vi "Remove Step.vi"(11 "Settings UI in":refnum<class "Settings UI.lvclass">) -> (3 "Settings UI out":refnum<class "Settings UI.lvclass">)   [LabVIEW 2020, in "Output Sequencer.lvlib" / "Settings UI.lvclass"]
uses:
  Settings UI.lvclass
  Settings UI.lvclass/Settings UI.ctl
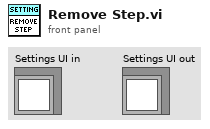
[diagram p1: front panel]
types:
  T1 = map{i32, cluster{"Step Number":i32, "Description":string}}
  T2 = typedef "Output Sequencer.lvlib/Settings UI.lvclass/Step Settings.ctl" = cluster{"Description":string, "Precondition":string, "Duration":dbl, "Mode":string, "Delay Between Values":dbl, "Analog Values":string[], "Digital Values":string[], "Postcondition":string, "On True":string, "On False":string}
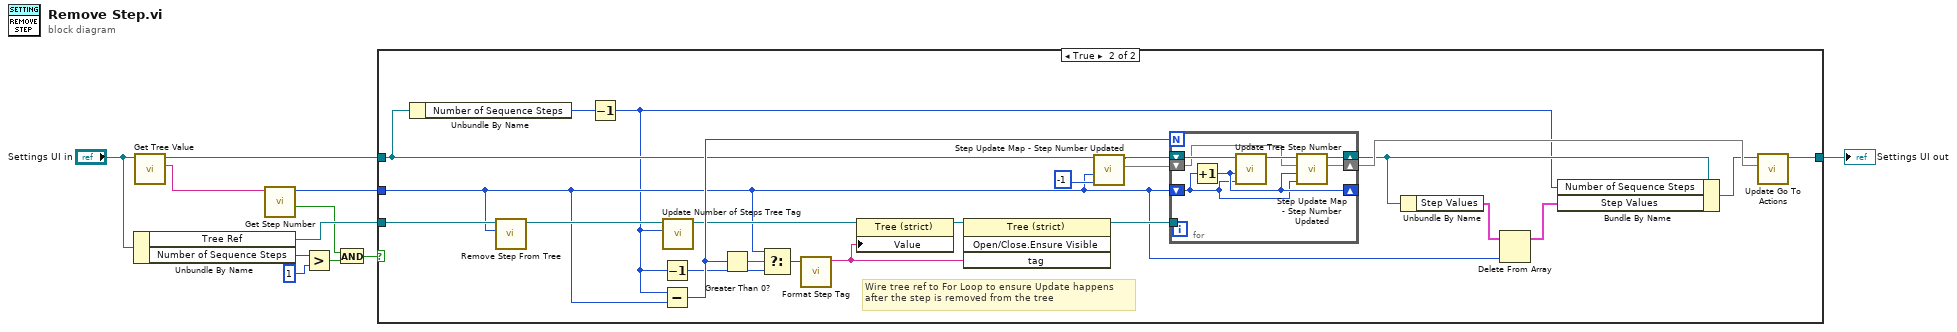
[diagram p0: block diagram]
diagram:
  n1 = Unbundle By Name("Settings UI in") -> ("Tree Ref"=w9:refnum<vi>, "Number of Sequence Steps"=w4:i32)
  n2 = call "Get Tree Value.vi"("UI Data in"="Settings UI in") -> ("Value"=w2:string, "UI Data out"=w10:refnum<class "Settings UI.lvclass">)  [unwired: 9 in]
  n3 = call "Get Step Number.vi"("Tree Tag"=w2) -> ("Is Step tag?"=w7:bool, "Step Number"=w3:i32)  [unwired: 8 in, 1 out]
  n4 = Greater?(x=w4, y=1) -> (0:w6:bool)
  n5 = And(x=w7, y=w6) -> (x .and. y?=w8:bool)
  n6 = case shown="True" w8 {
    tunnel: w3 -> [_ w15]
    tunnel: w10 -> [w12 w14]
    tunnel: [w12 w24] -> w11
    tunnel: w9 -> [_ w27]
    frame False {
    }
    frame True {
      # "Wire tree ref to For Loop to ensure Update happens\nafter the step is removed from the tree"
      n7 = Unbundle By Name(w14) -> ("Number of Sequence Steps"=w35:i32)
      n8 = call "Remove Step From Tree.vi"("Step Index"=w15, "TreeControl in"=w27) -> ("TreeControl out"=w34:refnum<vi>)  [unwired: 9 in]
      n9 = Decrement(x=w35) -> (x-1=w13:i32)
      n10 = Decrement(x=w13) -> (x-1=w31:i32)
      n11 = Subtract(x=w13, y=w15) -> (x-y=w33:i32)
      n12 = call "Update Number of Steps Tree Tag.vi"("New Number of Steps"=w13, "TreeControl in"=w34) -> ("TreeControl out"=w26:refnum<vi>)  [unwired: 9 in]
      n13 = Greater Than 0?(x=w33) -> (x > 0?=w32:bool)
      n14 = Select(t=w15, s=w32, f=w31) -> (s? t:f=w28:i32)
      n15 = call "Format Step Tag.vi"("Step Number"=w28) -> ("Tag"=w29:string)  [unwired: 10 in]
      n16 = property class="Tree (strict)"(reference=w26, "Value"=w29) -> (reference out=w30:refnum<vi>)  [unwired: 1 in, 1 out]
      n17 = invoke class="Tree (strict)" method="Open/Close.Ensure Visible"(reference=w30, "tag"=w29) -> (reference out=w25:refnum<vi>)  [unwired: 2 in, 3 out]
      n18 = call "Step Update Map - Step Number Updated.vi"("New Step Number"=-1, "Previous Step Number"=w15, "Settings UI in"=w14) -> ("Step Update Map out"=w20:T1, "Settings UI out"=w22:refnum<class "Settings UI.lvclass">)  [unwired: 7 in]
      n19 = for {
        N: w33 -> [_]
        shift-right: [w40] -> _
        shift-left: w15 -> [w38]
        shift-right: [w39] -> w19
        shift-left: w22 -> [w42]
        tunnel: w25 -> [_]
        shift-right: [w37] -> w23
        shift-left: w20 -> [w36]
        n20 = Increment(x=w38) -> (x+1=w40:i32)
        n21 = call "Update Tree Step Number.vi"("New Step Number"=w38, "Old Step Number"=w40, "UI Data In"=w42) -> ("UI Data Out"=w41:refnum<class "Settings UI.lvclass">)  [unwired: 6 in, 2 out]
        n22 = call "Step Update Map - Step Number Updated.vi"("New Step Number"=w38, "Previous Step Number"=w40, "Step Update Map in"=w36, "Settings UI in"=w41) -> ("Step Update Map out"=w37:T1, "Settings UI out"=w39:refnum<class "Settings UI.lvclass">)  [unwired: 6 in]
      }
      n23 = Unbundle By Name(w19) -> ("Step Values"=w17:T2[])
      n24 = Delete From Array(array=w17, index=w15) -> (array with subset deleted=w16:T2[])  [unwired: 1 in, 1 out]
      n25 = Bundle By Name(cluster=w19, "Number of Sequence Steps"=w13, "Step Values"=w16) -> (w18:refnum<class "Settings UI.lvclass">)
      n26 = call "Update Go To Actions.vi"("Step Update Map in"=w23, "Settings UI in"=w18) -> ("Settings UI out"=w24:refnum<class "Settings UI.lvclass">)  [unwired: 9 in]
    }
  }
  "Settings UI out" <- w11
